vi "parse_list_cameras.vi"(4 "error in":errorcluster, 7 "msg in":string="\u0000\u0003\u0000\u0000\u0000\u000b\u0000\u0000\u0000head_camera\u0010\u0000\u0000\u0000left_hand_camera\u0011\u0000\u0000\u0000right_hand_camera") -> (0 "error out":errorcluster, 2 "Cameras List":T1, 3 "msg out":string)   [LabVIEW 2012]
doc: "Parses a message into a list of cameras"
uses:
  std_msgs/subs/parse_u8_scalar.vi
  std_msgs/subs/parse_string_array.vi
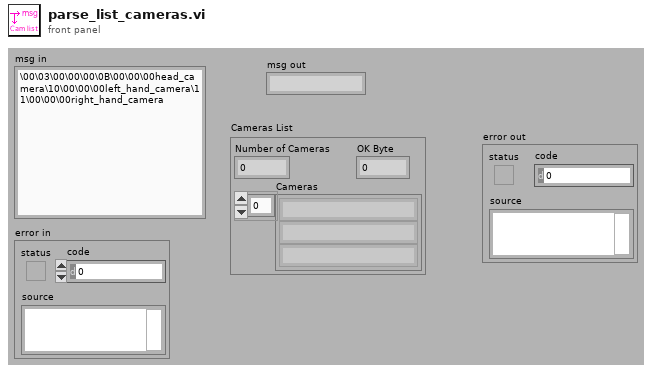
[diagram p1: front panel]
types:
  T1 = cluster{"Number of Cameras":i32, "Cameras":string[], "OK Byte":u8}
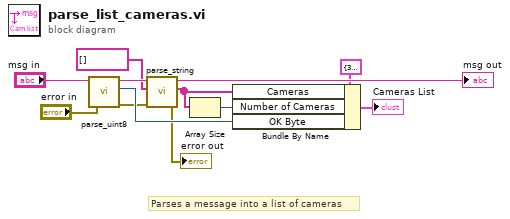
[diagram p0: block diagram]
diagram:
  # "Parses a message into a list of cameras"
  n1 = call-poly "parse_uint8.vi"("error in"="error in", "msg in"="msg in") -> ("error out"=w3:errorcluster, "number"=w7:u8, "msg out"=w6:string)  [unwired: 3 in]
  n2 = call-poly "parse_string.vi"("error in"=w3, "type"=string[] [] ("Cameras"), "msg in"=w6) -> ("error out"=→"error out":errorcluster, "strings"=w4:string[], "msg out"=→"msg out":string)  [unwired: 2 in]
  n3 = Array Size(array=w4) -> (size(s)=w8:i32)
  n4 = Bundle By Name(cluster=T1 {"Number of Cameras"=3, "Cameras"=["head_camera", "left_hand_camera", "right_hand_camera"], "OK Byte"=3} ("Cameras List"), "Cameras"=w4, "Number of Cameras"=w8, "OK Byte"=w7) -> (→"Cameras List":T1)
